vi "MAG_UI_Main.vi"() -> ()   [LabVIEW 2018]
doc: "Use this template to build a simple state machine design pattern. Each state executes code and determines which state to transition to."
uses:
  controls/MAG_UI_Data.ctl
  controls/MAG_UI_Command.ctl
  controls/MAG_Comms_State.ctl
  controls/Sensor_Data.ctl
  controls/BT_Devices.ctl
  <vilib>/Native 3D Graph/xcontrol/3DPC_SurfacePlot.xctl
  controls/MAG_UI_State.ctl
  controls/MAG_Display_State.ctl
  controls/MAG_UI_Comms_Config.ctl
  subVIs/calibration/FGVs/FGV States.ctl
panel:
  in  "Button_Sys_Check":bool
  in  "UI_Tab":T1(tab)
  out "Sensor Readings":dbl[][](array[numeric])=[[207.276, -3680.651, -5885.44], [494.158, -4382.085, -5575.68], [301.151, -4004.332, -4646.4], [401.034, -4427.145, -4646.4], [87.867, -4272.439, -4646.4], [-42.056, -4150.777, -4026.88], [-226.802, -4030.617, -3407.3599999999997], [225.3, -4882.251, -4026.88], [349.966, -3422.307, -5575.68], [254.589, -3876.662, -5575.68], [485.897, -4172.556, -4646.4], [107.393, -3751.245, -4026.88], [97.63, -4424.141, -3717.12], [-0.751, -4374.575, -4026.88], [-150.951, -3895.437, -4026.88], [-451.351, -4812.408, -4336.639999999999], [-148.698, -3219.537, -5885.44], [120.911, -4482.719, -5885.44], [-244.826, -3894.686, -4646.4], [-131.425, -3897.69, -4026.88], [-337.95, -4164.295, -4336.639999999999], [-461.865, -4094.452, -4336.639999999999], [-414.552, -3842.116, -4336.639999999999], [-774.281, -5015.929, -4646.4], [-63.084, -4473.707, -5885.44], [-47.313, -3474.126, -5265.92], [-464.869, -4331.017, 4026.88], [-458.11, -4048.641, -4646.4], [-462.616, -4204.849, -4336.639999999999], [-644.358, -4587.108, -5265.92], [-526.451, -4170.303, -4646.4], [-1116.737, -5181.9, -4956.16], [316.922, -4416.631, -5885.44], [-174.983, -3826.345, -5885.44], [-693.924, -3861.642, -4646.4], [-112.65, -4486.474, -4646.4], [-210.28, -3921.722, -4956.16], [-518.19, -4052.396, -4956.16], [-841.871, -4038.127, -4956.16], [-1354.804, -4737.308, -4956.16], [-153.204, -3745.988, -6195.2], [181.742, -3714.446, -5885.44], [0.751, 0.751, 309.76], [-799.064, -4349.041, -4956.16], [-1019.858, -4024.609, -5265.92], [-565.503, -4018.601, -5265.92], [-770.526, -4175.56, -5575.68], [-1125.749, -5006.166, -5575.68], [496.411, -4216.114, -7124.48], [-14.269, -3723.458, -6504.96], [-910.963, -4006.585, -6195.2], [-1396.86, -4133.504, -5575.68], [-1124.247, -4031.368, -4646.4], [-1948.094, -3513.929, -6195.2], [-1823.428, -3645.354, -5575.68], [-2681.07, -4476.711, -5885.44], [-389.018, -2473.794, -5575.68], [-982.308, -2724.628, -6195.2], [-1058.91, -2711.11, -5575.68], [-1121.994, -2741.15, 4956.16], [-1360.812, -3184.991, 2168.3199999999997], [-2020.941, -4083.187, -5575.68], [-1991.652, -3568.001, -5575.68], [-1966.869, -4436.908, -6195.2]]
  in  "Tab Control":enum32{"2D", "3D"}(tab)=enum."3D"
  out "Node Response":T2(graph)
  in  "Node":i32
  out "3D Graph":refnum<class "Base Datatype.lvclass">[](xcontrol)
  in  "Logfile Store":path
  in  "Get File":bool
  in  "Stop Logging":bool
  out "Elapsed Samples":i32
  in  "Log File ID":string
  out "File System Information":string
  in  "Comms Setting":enum32{"Serial", "Bluetooth"}(tab)=enum."Bluetooth"
  in  "VISA resource name":refnum<visa-resource-name>="COM11"
  in  "Serial Settings":T3={"baud rate"=115200, "data bits"=8, "parity"=enum."None", "stop bits"=10, "flow control"=0} {"flow control" items=["None"=0, "XON/XOFF"=1, "RTS/CTS"=2, "DTR/DSR"=4]; "stop bits" items=["1.0"=10, "1.5"=15, "2.0"=20]; "data bits" min=5 max=8 step=1; "baud rate" items=["75"=75, "110"=110, "134"=134, "150"=150, "300"=300, "600"=600, "1200"=1200, "1800"=1800, "2400"=2400, "4800"=4800, "7200"=7200, "9600"=9600, "14400"=14400, "19200"=19200, "28800"=28800, "38400"=38400, "56000"=56000, "57600"=57600, "115200"=115200, "128000"=128000, "230400"=230400]}
  in  "BT address":string="00:14:03:05:08:37"
  in  "BT Channel (0)":u16=1
  in  "Calibration File":string="6x0-5mm"
  out "Comm State":T4
  out "notification":T6
  out "comms":i32=1114490
  out "ui":i32=2866
  out "Comm Er":errorcluster={"status"=TRUE, "code"=1, "source"="Wait on Notification in MAG_UI_Main.vi"}
  out "Available BT Devices":T7
  in  "Discover BT Devices":bool
  in  "Button_Disconnect":bool
  in  "Button_Initialise":bool
  in  "Button_Stream":bool
  out "Status":T8={"System Version"="", "Connected"=TRUE, "Active?"=TRUE, "Streaming"=TRUE, "Logging"=FALSE}
  in  "Button_Record":bool
  in  "Button_Connect":bool
  in  "Button_Exit":bool
  # "ESCAPES"
  # "Select this tab to use Direct Bluetooth connectivity"
  # "20:16:12:12:64:24"
  # "00:06:66:8c:9e:7d"
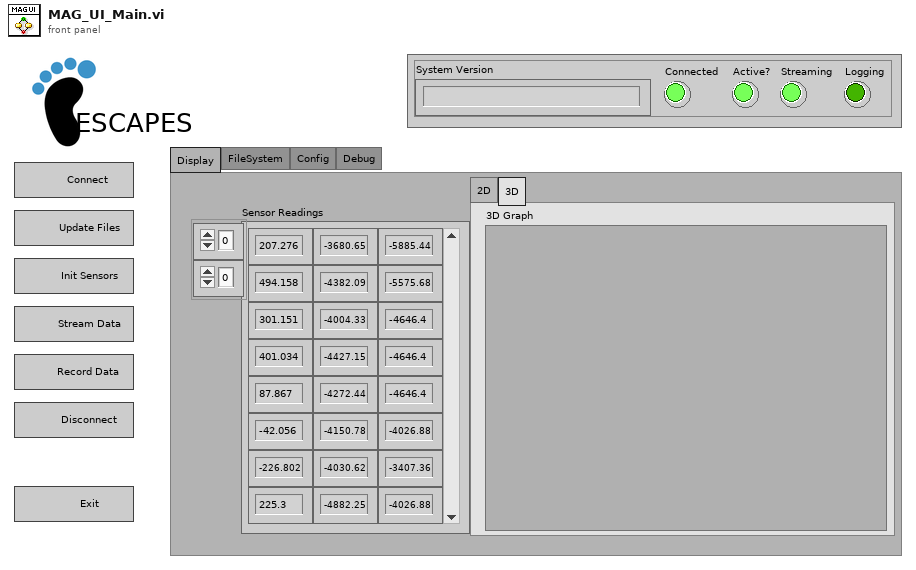
[diagram p1: front panel]
types:
  T1 = enum32{"Display", "FileSystem", "Config", "Debug"}
  T2 = cluster{"Node XYZ List[0]":dbl, "Node XYZ List[1]":dbl, "Node XYZ List[2]":dbl}
  T3 = cluster{"baud rate":u32, "data bits":u16, "parity":enum16{"None", "Odd", "Even", "Mark", "Space"}, "stop bits":u16, "flow control":u16}
  T4 = typedef "MAG_UI_Command.ctl" = cluster{"Comms_States":T5, "Parameters":string, "Clear Buffer?":bool}
  T5 = typedef "MAG_Comms_State.ctl" = enum16{"Initialize", "Wait for Event", "Connect", "Send_Com", "Rcv_TXT", "Rcv_BIN", "Rcv_FILE", "Disconnect"}
  T6 = typedef "Sensor_Data.ctl" = cluster{"Time":u32, "Data":dbl[][]}
  T7 = typedef "BT_Devices.ctl" = cluster{"Address":string, "Device Name":string}[]
  T8 = typedef "MAG_UI_Data.ctl" = cluster{"System Version":string, "Connected":bool, "Active?":bool, "Streaming":bool, "Logging":bool}
  T9 = typedef "MAG_UI_Comms_Config.ctl" = cluster{enum16{"Serial", "Bluetooth"}, "Serial Refnum":refnum<visa-resource-name>, "BT ID":refnum<k31>}
  T10 = typedef "MAG_Display_State.ctl" = enum16{"Initialise", "Display", "Exit"}
  T11 = typedef "MAG_UI_State.ctl" = enum16{"Initialize", "Wait for Event", "Com_Connect", "Com_Init_Sys", "Com_Chk_Sys", "Com_Stream", "Com_Log", "Com_Get", "Exit"}
  T12 = typedef "FGV States.ctl" = enum16{"Get", "Set", "Reset"}
  T13 = cluster{cluster{dbl[][], "Array":dbl[][]}, cluster{dbl[][], "Array":dbl[][]}, cluster{dbl[][], "Array":dbl[][]}, cluster{dbl[][], "Array":dbl[][]}}
  T14 = cluster{cluster{dbl[][], "Array":dbl[][]}, cluster{dbl[][], "Array":dbl[][]}, cluster{dbl[][], "Array":dbl[][]}, cluster{dbl[][], "Array":dbl[][]}}[]
  T15 = cluster{"Mag_GRID[0]":dbl, "Mag_GRID[1]":dbl, "Mag_GRID[2]":dbl}
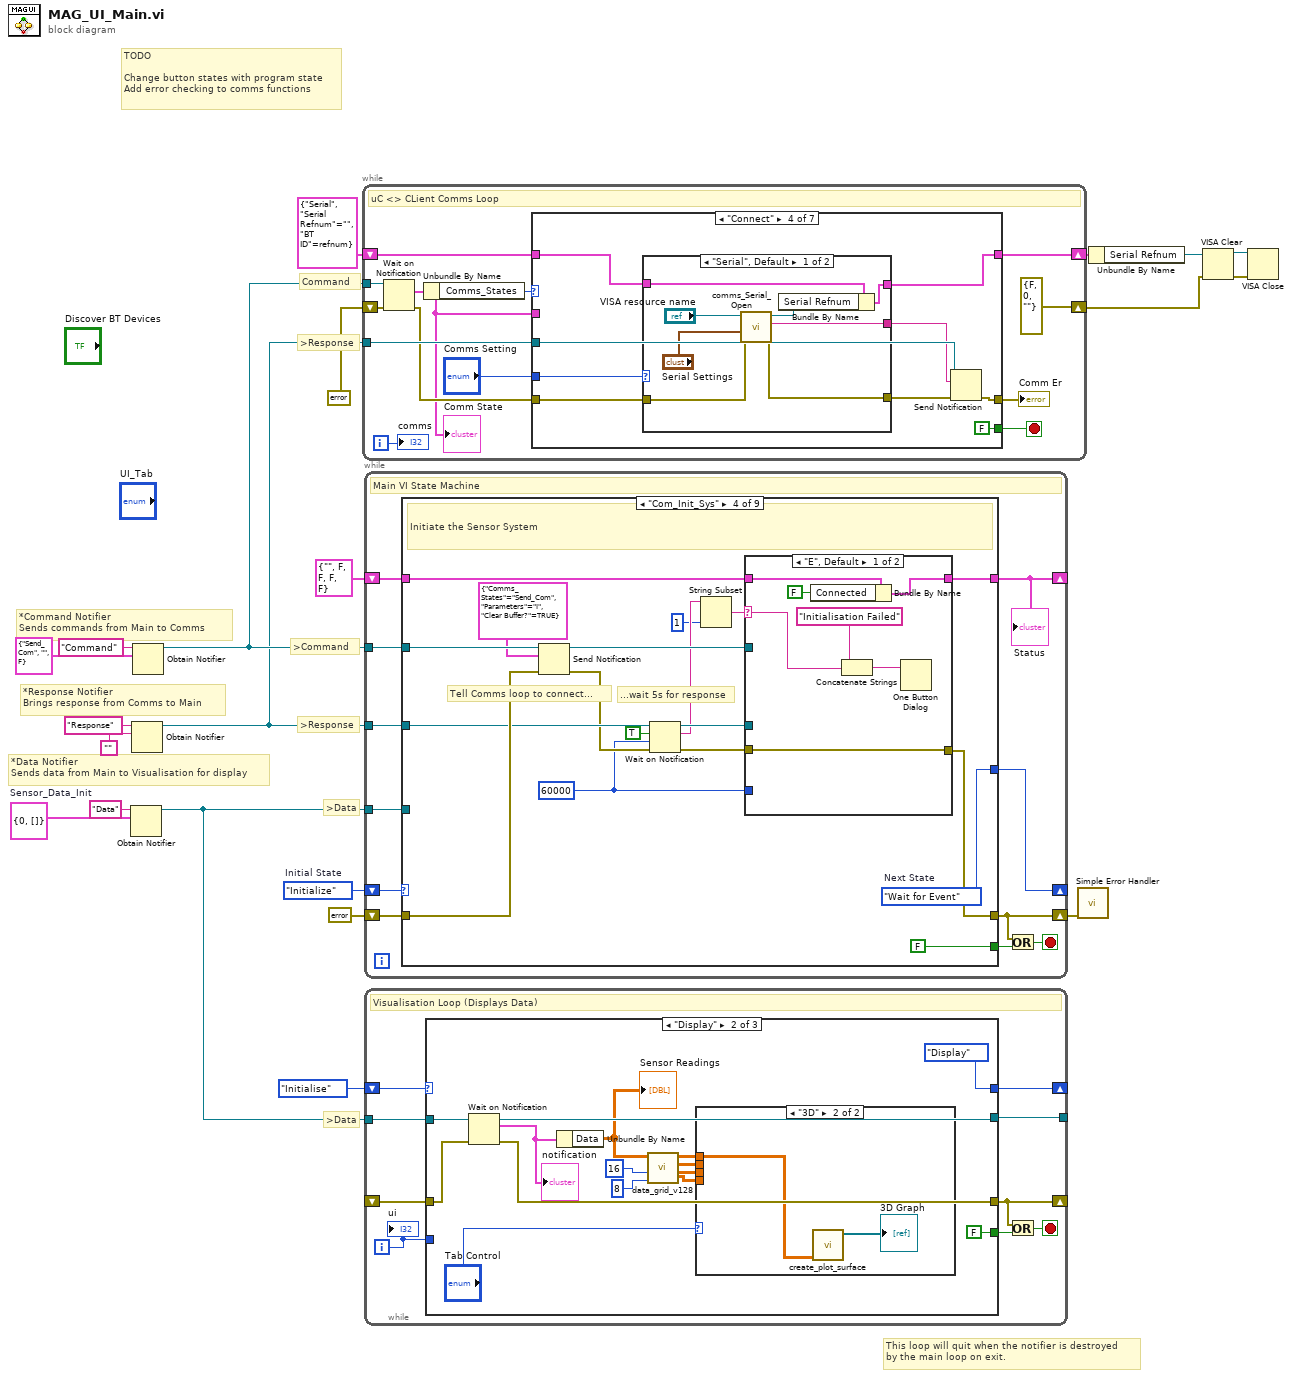
[diagram p0: block diagram]
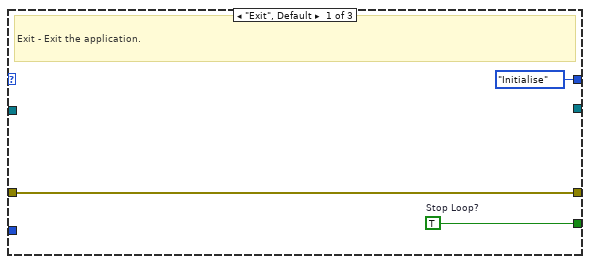
[diagram p2: hidden frame]
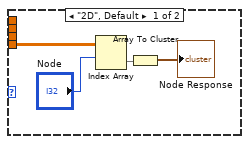
[diagram p3: hidden frame]
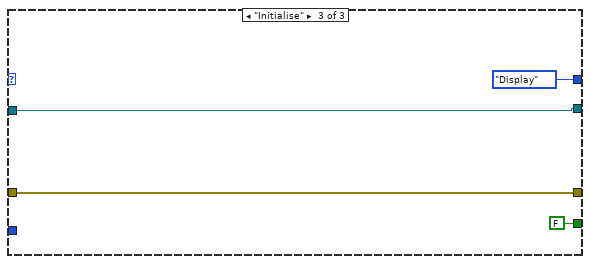
[diagram p4: hidden frame]
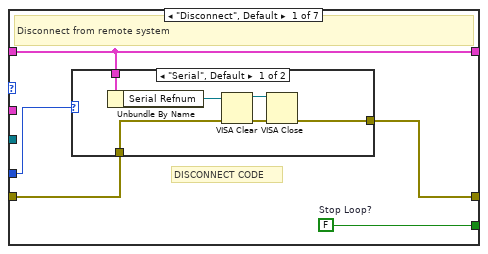
[diagram p5: hidden frame]
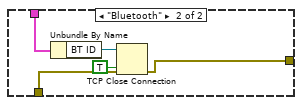
[diagram p6: hidden frame]
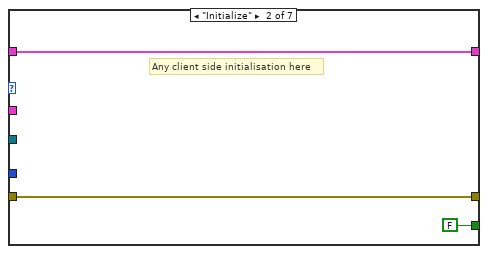
[diagram p7: hidden frame]
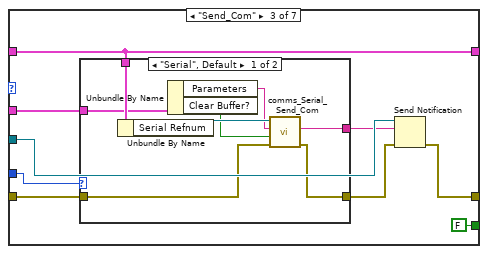
[diagram p8: hidden frame]
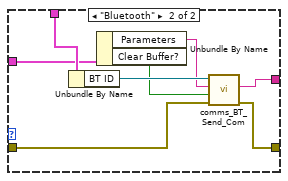
[diagram p9: hidden frame]
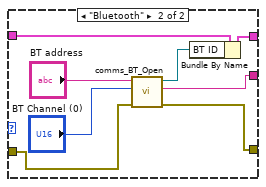
[diagram p10: hidden frame]
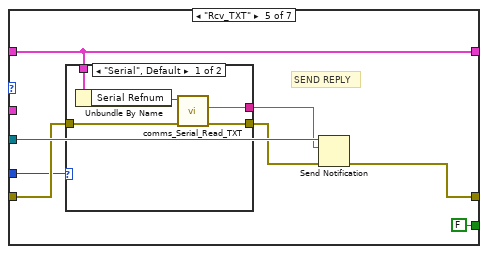
[diagram p11: hidden frame]
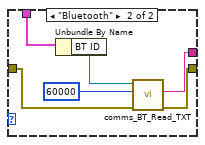
[diagram p12: hidden frame]
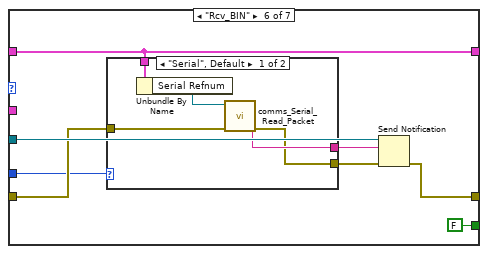
[diagram p13: hidden frame]
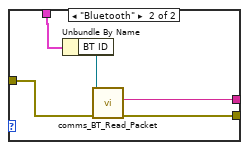
[diagram p14: hidden frame]
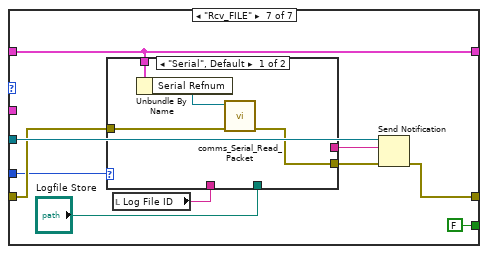
[diagram p15: hidden frame]
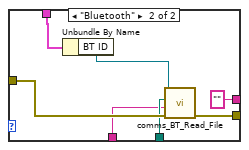
[diagram p16: hidden frame]
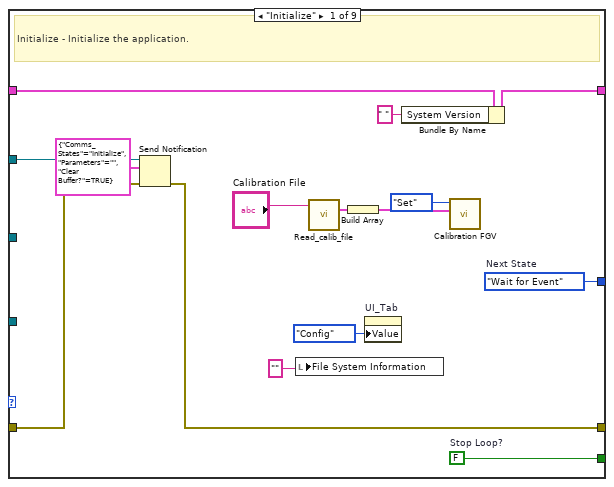
[diagram p17: hidden frame]
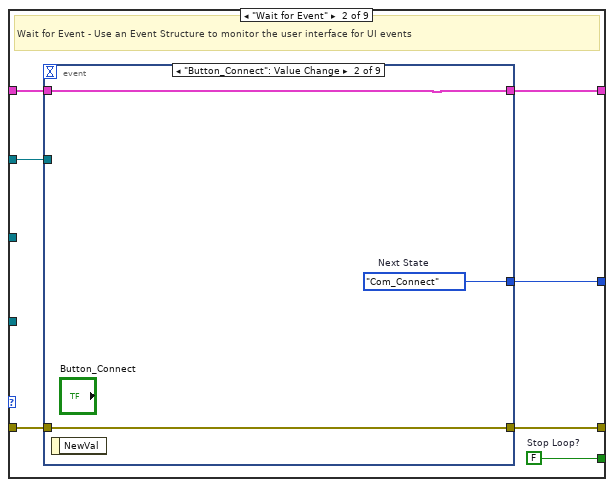
[diagram p18: hidden frame]
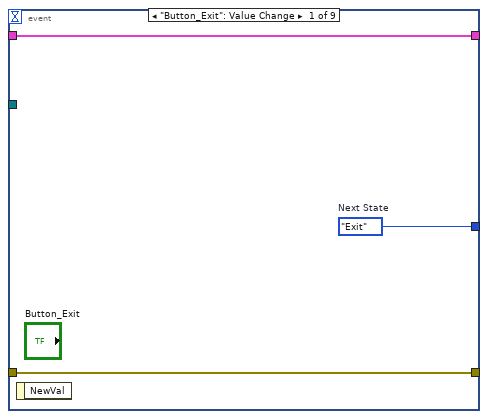
[diagram p19: hidden frame]
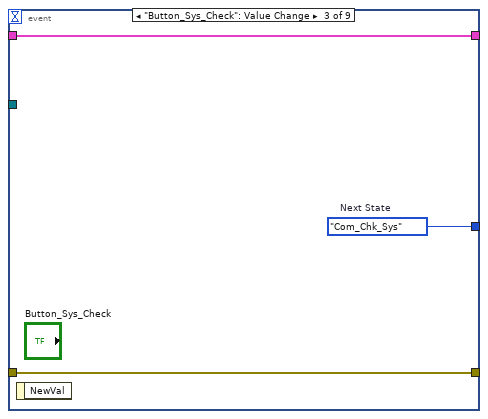
[diagram p20: hidden frame]
diagram:
  w10 = T6 {"Time"=0, "Data"=[]}  # Sensor_Data_Init
  w21 = MAG_UI_State."Initialize"  # Initial State
  # "TODO\n\nChange button states with program state\nAdd error checking to comms functions"
  # "This loop will quit when the notifier is destroyed\nby the main loop on exit."
  # ">Data"
  # ">Data"
  # ">Response"
  # ">Response"
  # ">Command"
  # "*Data Notifier\nSends data from Main to Visualisation for display"
  # "*Response Notifier\nBrings response from Comms to Main"
  # "*Command Notifier\nSends commands from Main to Comms"
  # "Command"
  n1 = Obtain Notifier(name (unnamed)="Data", notification data type=w10) -> (notifier out=w12:refnum<notifier>)  [unwired: 2 in, 2 out]
  n2 = Obtain Notifier(name (unnamed)="Response", notification data type="") -> (notifier out=w11:refnum<notifier>)  [unwired: 2 in, 2 out]
  n3 = Obtain Notifier(name (unnamed)="Command", notification data type=T4 {"Comms_States"=enum."Send_Com", "Parameters"="", "Clear Buffer?"=FALSE}) -> (notifier out=w15:refnum<notifier>)  [unwired: 2 in, 2 out]
  n4 = while {
    shift-right: [errorcluster {"status"=FALSE, "code"=0, "source"=""} ("error constant")] -> w1
    shift-left: errorcluster {"status"=FALSE, "code"=0, "source"=""} ("error constant") -> [w30]
    tunnel: w15 -> [w32]
    tunnel: w11 -> [w34]
    shift-right: [w27] -> w2
    shift-left: T9 {enum."Serial", "Serial Refnum"="", "BT ID"=refnum} -> [w28]
    i -> [w26]
    stop <- w24 stop-if-true
    # "uC <> CLient Comms Loop"
    n5 = Wait on Notification(notifier=w32, error in (no error)=w30) -> (notification=w25:T4, error out=w29:errorcluster)  [unwired: 2 in, 2 out]
    "Comm State" <- w25
    n6 = Unbundle By Name(w25) -> ("Comms_States"=w31:T5)
    n7 = case shown="\"Connect\"" w31 {
      tunnel: [w39 FALSE ("Stop Loop?") FALSE ("Stop Loop?") FALSE ("Stop Loop?") FALSE ("Stop Loop?") FALSE ("Stop Loop?") FALSE ("Stop Loop?")] -> w24
      tunnel: w29 -> [w38 w52 w57 w81 w107 w125 w145]
      tunnel: [w37 w52 w61 w87 w110 w129 w149] -> w33
      tunnel: w34 -> [_ _ w62 w85 w111 w128 w148]
      tunnel: w28 -> [w36 w51 w58 w83 w108 w126 w146]
      tunnel: [w36 w51 w58 w82 w108 w126 w146] -> w27
      tunnel: w25 -> [_ _ w55 _ _ _ _]
      tunnel: "Comms Setting" -> [w35 _ w54 w79 w104 w123 w143]
      frame "Disconnect", Default {
        w39 = FALSE  # Stop Loop?
        # "DISCONNECT CODE"
        # "Disconnect from remote system"
        n8 = case shown="\"Serial\", Default" w35 {
          tunnel: w38 -> [w42 w48]
          tunnel: [w41 w47] -> w37
          tunnel: w36 -> [w40 w50]
          frame "Serial", Default {
            n9 = Unbundle By Name(w40) -> ("Serial Refnum"=w45:refnum<visa-resource-name>)
            n10 = VISA Clear(VISA resource name=w45, error in (no error)=w42) -> (VISA resource name out=w43:refnum<visa-resource-name>, error out=w44:errorcluster)
            n11 = VISA Close(VISA resource name=w43, error in (no error)=w44) -> (error out=w41:errorcluster)
          }
          frame "Bluetooth" {
            n12 = Unbundle By Name(w50) -> ("BT ID"=w49:refnum<k31>)
            n13 = TCP Close Connection(connection ID=w49, abort (F)=TRUE, error in (no error)=w48) -> (error out=w47:errorcluster)  [unwired: 1 out]
          }
        }
      }
      frame "Initialize" {
        # "Any client side initialisation here"
      }
      frame "Send_Com" {
        n14 = case shown="\"Serial\", Default" w54 {
          tunnel: [w69 w71] -> w59
          tunnel: w58 -> [w68 w78]
          tunnel: w57 -> [w67 w76]
          tunnel: [w66 w75] -> w56
          tunnel: w55 -> [w64 w77]
          frame "Serial", Default {
            n15 = Unbundle By Name(w68) -> ("Serial Refnum"=w70:refnum<visa-resource-name>)
            n16 = Unbundle By Name(w64) -> ("Parameters"=w63:string, "Clear Buffer?"=w65:bool)
            n17 = call "comms_Serial_Send_Com.vi"("error in"=w67, "Buffer Clear?"=w65, "Command"=w63, "VISA resource in"=w70) -> ("error out"=w66:errorcluster, "Response"=w69:string)  [unwired: 5 in, 1 out]
          }
          frame "Bluetooth" {
            n18 = Unbundle By Name(w78) -> ("BT ID"=w74:refnum<k31>)
            n19 = Unbundle By Name(w77) -> ("Parameters"=w73:string, "Clear Buffer?"=w72:bool)
            n20 = call "comms_BT_Send_Com.vi"("error in"=w76, "Buffer Clear?"=w72, "Command"=w73, "connection ID"=w74) -> ("error out"=w75:errorcluster, "Response"=w71:string)  [unwired: 5 in, 1 out]
          }
        }
        n21 = Send Notification(notification=w59, notifier=w62, error in (no error)=w56) -> (error out=w61:errorcluster)  [unwired: 1 out]
      }
      frame "Connect" {
        n22 = case shown="\"Serial\", Default" w79 {
          tunnel: [w89 w100] -> w84
          tunnel: w83 -> [w93 w99]
          tunnel: [w91 w97] -> w82
          tunnel: w81 -> [w90 w101]
          tunnel: [w88 w96] -> w80
          frame "Serial", Default {
            n23 = call "comms_Serial_Open.vi"("error in (no error)"=w90, "Serial Settings in"="Serial Settings", "VISA Refnum in"="VISA resource name") -> ("error out"=w89:errorcluster, "Data Out"=w88:string, "VISA Refnum out"=w92:refnum<visa-resource-name>)  [unwired: 6 in]
            n24 = Bundle By Name(cluster=w93, "Serial Refnum"=w92) -> (w91:T9)
          }
          frame "Bluetooth" {
            n25 = call "comms_BT_Open.vi"("error in (no error)"=w101, "BT Channel (0)"="BT Channel (0)", "BT address"="BT address") -> ("error out"=w100:errorcluster, "Response"=w96:string, "Bluetooth Network Connection out"=w98:refnum<k31>)  [unwired: 6 in]
            n26 = Bundle By Name(cluster=w99, "BT ID"=w98) -> (w97:T9)
          }
        }
        n27 = Send Notification(notification=w80, notifier=w85, error in (no error)=w84) -> (error out=w87:errorcluster)  [unwired: 1 out]
      }
      frame "Rcv_TXT" {
        # "SEND REPLY"
        n28 = case shown="\"Serial\", Default" w104 {
          tunnel: w108 -> [w116 w122]
          tunnel: w107 -> [w114 w118]
          tunnel: [w113 w119] -> w106
          tunnel: [w112 w120] -> w105
          frame "Serial", Default {
            n29 = Unbundle By Name(w116) -> ("Serial Refnum"=w115:refnum<visa-resource-name>)
            n30 = call "comms_Serial_Read_TXT.vi"("error in"=w114, "VISA resource in"=w115) -> ("error out"=w113:errorcluster, "Data Out"=w112:string)  [unwired: 6 in, 2 out]
          }
          frame "Bluetooth" {
            n31 = Unbundle By Name(w122) -> ("BT ID"=w121:refnum<k31>)
            n32 = call "comms_BT_Read_TXT.vi"("error in"=w118, "timeout ms (25000)"=60000, "connection ID"=w121) -> ("error out"=w119:errorcluster, "Data Out"=w120:string)  [unwired: 5 in, 2 out]
          }
        }
        n33 = Send Notification(notification=w105, notifier=w111, error in (no error)=w106) -> (error out=w110:errorcluster)  [unwired: 1 out]
      }
      frame "Rcv_BIN" {
        n34 = case shown="\"Serial\", Default" w123 {
          tunnel: [w135 w136] -> w127
          tunnel: w126 -> [w133 w140]
          tunnel: w125 -> [w132 w138]
          tunnel: [w131 w137] -> w124
          frame "Serial", Default {
            n35 = Unbundle By Name(w133) -> ("Serial Refnum"=w134:refnum<visa-resource-name>)
            n36 = call "comms_Serial_Read_Packet.vi"("error in"=w132, "VISA resource in"=w134) -> ("error out"=w131:errorcluster, "Data Out"=w135:string)  [unwired: 6 in, 2 out]
          }
          frame "Bluetooth" {
            n37 = Unbundle By Name(w140) -> ("BT ID"=w139:refnum<k31>)
            n38 = call "comms_BT_Read_Packet.vi"("error in"=w138, "connection ID"=w139) -> ("error out"=w137:errorcluster, "Data Out"=w136:string)  [unwired: 7 in, 1 out]
          }
        }
        n39 = Send Notification(notification=w127, notifier=w128, error in (no error)=w124) -> (error out=w129:errorcluster)  [unwired: 1 out]
      }
      frame "Rcv_FILE" {
        n40 = local read "Log File ID"() -> (w141:string)
        n41 = case shown="\"Serial\", Default" w143 {
          tunnel: [_ "" ("source")] -> w147
          tunnel: w146 -> [w153 w161]
          tunnel: w145 -> [w152 w159]
          tunnel: [w151 w158] -> w144
          tunnel: "Logfile Store" -> [_ w156]
          tunnel: w141 -> [_ w155]
          frame "Serial", Default {
            n42 = Unbundle By Name(w153) -> ("Serial Refnum"=w154:refnum<visa-resource-name>)
            n43 = call "comms_Serial_Read_Packet.vi"("error in"=w152, "VISA resource in"=w154) -> ("error out"=w151:errorcluster)  [unwired: 6 in, 3 out]
          }
          frame "Bluetooth" {
            n44 = Unbundle By Name(w161) -> ("BT ID"=w160:refnum<k31>)
            n45 = call "comms_BT_Read_File.vi"("error in"=w159, "filename"=w155, "file path (use dialog)"=w156, "connection ID"=w160) -> ("error out"=w158:errorcluster)  [unwired: 6 in, 1 out]
          }
        }
        n46 = Send Notification(notification=w147, notifier=w148, error in (no error)=w144) -> (error out=w149:errorcluster)  [unwired: 1 out]
      }
    }
    "Comm Er" <- w33
    "comms" <- w26
  }
  n47 = while {
    shift-right: [w171] -> _
    shift-left: w21 -> [w172]
    shift-right: [w162] -> _
    shift-left: T8 {"System Version"="", "Connected"=FALSE, "Active?"=FALSE, "Streaming"=FALSE, "Logging"=FALSE} ("Data") -> [w170]
    shift-right: [w166] -> w18
    shift-left: errorcluster {"status"=FALSE, "code"=0, "source"=""} ("error constant") -> [w169]
    tunnel: w15 -> [w165]
    tunnel: w11 -> [w164]
    tunnel: w12 -> [w163]
    stop <- w167 stop-if-true
    # "Main VI State Machine"
    n48 = case shown="\"Com_Init_Sys\"" w172 {
      tunnel: [w187 w194 w248 w267 w305 w340 w376 w420 w462] -> w171
      tunnel: [w186 w193 FALSE ("Stop Loop?") FALSE ("Stop Loop?") FALSE ("Stop Loop?") FALSE ("Stop Loop?") FALSE ("Stop Loop?") FALSE ("Stop Loop?") w460] -> w168
      tunnel: w170 -> [w185 w192 w240 w271 w308 w344 w380 w423 w461]
      tunnel: [w184 w191 w239 w270 w307 w343 w379 w422 w461] -> w162
      tunnel: w169 -> [w180 w190 w245 w274 w311 w347 w383 w426 w456]
      tunnel: [w179 w189 w242 w264 w302 w337 w373 w417 w455] -> w166
      tunnel: w165 -> [w182 w188 w246 w275 w312 w348 w384 w427 w459]
      tunnel: w164 -> [_ _ w244 w273 w310 w346 w382 w425 w453]
      tunnel: w163 -> [_ _ _ _ _ _ w369 w413 w452]
      frame "Initialize" {
        w186 = FALSE  # Stop Loop?
        w187 = MAG_UI_State."Wait for Event"  # Next State
        # "Initialize - Initialize the application."
        n49 = Send Notification(notification=T4 {"Comms_States"=enum."Initialize", "Parameters"="", "Clear Buffer?"=TRUE}, notifier=w182, error in (no error)=w180) -> (error out=w179:errorcluster)  [unwired: 1 out]
        n50 = local write "File System Information"("" ("File System Information")) -> ()
        n51 = call "Read_calib_file.vi"("string"="Calibration File") -> ("output cluster"=w175:T13)  [unwired: 6 in, 4 out]
        n52 = Build Array(w175) -> (w174:T14)
        n53 = property on="UI_Tab" class="TabCtl (strict)"("Value"=T1."Config" ("UI_Tab")) -> ()  [unwired: 2 in, 2 out]
        n54 = Bundle By Name(cluster=w185, "System Version"=" ") -> (w184:T8)
        n55 = call "Calibration FGV.vi"("Calib in"=w174, "FGV States"=FGV_States."Set") -> ()  [unwired: 9 in, 1 out]
      }
      frame "Wait for Event" {
        w193 = FALSE  # Stop Loop?
        # "Wait for Event - Use an Event Structure to monitor the user interface for UI events"
        n56 = event shown="[1] \"Button_Connect\": Value Change" {
          selector: _ -> [_ _ _ _ _ _ _ _ _]
          dyn-events: _ -> [_ _ _ _ _ _ _ _ _]
          timeout: _ -> [_ _ _ _ _ _ _ _ _]
          tunnel: [w197 w200 w203 MAG_UI_State."Com_Init_Sys" ("Next State") MAG_UI_State."Com_Stream" ("Next State") MAG_UI_State."Wait for Event" ("Next State") MAG_UI_State."Com_Log" ("Next State") MAG_UI_State."Com_Get" ("Next State") MAG_UI_State."Wait for Event" ("Next State")] -> w194
          tunnel: w192 -> [w196 w198 w201 w206 w209 w215 w217 w223 w230]
          tunnel: [w196 w198 w201 w206 w208 w215 w216 w223 w229] -> w191
          tunnel: w190 -> [w195 w199 w202 w205 w211 w214 w220 w222 w232]
          tunnel: [w195 w199 w202 w205 w211 w214 w220 w222 w226] -> w189
          tunnel: w188 -> [_ _ _ _ _ _ _ _ w233]
          event "Button_Exit": Value Change {
            w197 = MAG_UI_State."Exit"  # Next State
            n57 = event-data() -> ()  [unwired: 1 in, 1 out]
          }
          event "Button_Connect": Value Change {
            w200 = MAG_UI_State."Com_Connect"  # Next State
            n58 = event-data() -> ()  [unwired: 1 in, 1 out]
          }
          event "Button_Sys_Check": Value Change {
            w203 = MAG_UI_State."Com_Chk_Sys"  # Next State
            n59 = event-data() -> ()  [unwired: 1 in, 1 out]
          }
          event "Button_Initialise": Value Change {
            n60 = event-data() -> ()  [unwired: 1 in, 1 out]
          }
          event "Button_Stream": Value Change {
            n61 = event-data() -> ()  [unwired: 1 in, 1 out]
            n62 = Bundle By Name(cluster=w209, "Streaming"=TRUE) -> (w208:T8)
          }
          event "Discover BT Devices": Value Change {
            n63 = event-data() -> ()  [unwired: 1 in, 1 out]
            n64 = call "BT_Discover.vi"() -> ("Active_BT_Devices"=→"Available BT Devices":T7)  [unwired: 11 in]
          }
          event "Button_Record": Value Change {
            n65 = event-data() -> ()  [unwired: 1 in, 1 out]
            n66 = Bundle By Name(cluster=w217, "Logging"=TRUE ("Streaming")) -> (w216:T8)
          }
          event "Get File": Value Change {
            n67 = event-data() -> ()  [unwired: 1 in, 1 out]
          }
          event "Button_Disconnect": Value Change {
            n68 = event-data() -> ()  [unwired: 1 in, 1 out]
            n69 = Send Notification(notification=T4 {"Comms_States"=enum."Send_Com", "Parameters"="X", "Clear Buffer?"=TRUE}, notifier=w233, error in (no error)=w232) -> (notifier out=w224:refnum<notifier>, error out=w227:errorcluster)
            n70 = Send Notification(notification=T4 {"Comms_States"=enum."Disconnect", "Parameters"="X", "Clear Buffer?"=TRUE}, notifier=w224, error in (no error)=w227) -> (error out=w226:errorcluster)  [unwired: 1 out]
            n71 = Bundle By Name(cluster=w230, "System Version"="") -> (w229:T8)
          }
        }
      }
      frame "Com_Connect" {
        w248 = MAG_UI_State."Wait for Event"  # Next State
        # "...wait 5s for response"
        # "Tell Comms loop to connect..."
        # "Connect to the System"
        n72 = Send Notification(notification=T4 {"Comms_States"=enum."Connect", "Parameters"="", "Clear Buffer?"=TRUE}, notifier=w246, error in (no error)=w245) -> (error out=w243:errorcluster)  [unwired: 1 out]
        n73 = Wait on Notification(notifier=w244, timeout in ms (-1)=5000, error in (no error)=w243) -> (notification=w235:string, error out=w242:errorcluster)  [unwired: 1 in, 2 out]
        n74 = String Subset(string=w235, length (rest)=1 ("offset (0)")) -> (substring=w237:string)  [unwired: 1 in]
        n75 = case shown="\"!\", Default" w237 {
          tunnel: w240 -> [w252 w256]
          tunnel: [w251 w255] -> w239
          tunnel: w235 -> [w249 w253]
          frame "!", Default {
            n76 = Bundle By Name(cluster=w252, "Connected"=TRUE, "System Version"=w249) -> (w251:T8)
          }
          frame "E" {
            n77 = Bundle By Name(cluster=w256, "Connected"=FALSE) -> (w255:T8)
            n78 = Concatenate Strings("Connection Error", w253) -> (w258:string)
            n79 = One Button Dialog(message=w258) -> ()  [unwired: 1 in, 1 out]
          }
        }
      }
      frame "Com_Init_Sys" {
        w267 = MAG_UI_State."Wait for Event"  # Next State
        w266 = 60000 ("timeout in ms (-1)")
        # "...wait 5s for response"
        # "Tell Comms loop to connect..."
        # "Initiate the Sensor System"
        n80 = Send Notification(notification=T4 {"Comms_States"=enum."Send_Com", "Parameters"="I", "Clear Buffer?"=TRUE}, notifier=w275, error in (no error)=w274) -> (notifier out=w268:refnum<notifier>, error out=w272:errorcluster)
        n81 = Wait on Notification(notifier=w273, ignore previous (F)=TRUE, timeout in ms (-1)=w266, error in (no error)=w272) -> (notifier out=w263:refnum<notifier>, notification=w260:string, error out=w265:errorcluster)  [unwired: 1 out]
        n82 = String Subset(string=w260, length (rest)=1 ("offset (0)")) -> (substring=w261:string)  [unwired: 1 in]
        n83 = case shown="\"E\", Default" w261 {
          selector: w261 -> [w281 _]
          tunnel: w271 -> [w280 w287]
          tunnel: [w279 w286] -> w270
          tunnel: w268 -> [_ w294]
          tunnel: w266 -> [_ w293]
          tunnel: w265 -> [w277 w292]
          tunnel: [w277 w290] -> w264
          tunnel: w263 -> [_ w289]
          frame "E", Default {
            n84 = Bundle By Name(cluster=w280, "Connected"=FALSE) -> (w279:T8)
            n85 = Concatenate Strings("Initialisation Failed", w281) -> (w283:string)
            n86 = One Button Dialog(message=w283) -> ()  [unwired: 1 in, 1 out]
          }
          frame "i" {
            n87 = Send Notification(notification=T4 {"Comms_States"=enum."Rcv_TXT", "Parameters"="", "Clear Buffer?"=FALSE}, notifier=w294, error in (no error)=w292) -> (error out=w291:errorcluster)  [unwired: 1 out]
            n88 = Bundle By Name(cluster=w287, "Active?"=TRUE) -> (w286:T8)
            n89 = Wait on Notification(notifier=w289, ignore previous (F)=TRUE, timeout in ms (-1)=w293, error in (no error)=w291) -> (notification=w284:string, error out=w290:errorcluster)  [unwired: 2 out]
            n90 = One Button Dialog(message=w284) -> ()  [unwired: 1 in, 1 out]
          }
        }
      }
      frame "Com_Get" {
        w305 = MAG_UI_State."Wait for Event"  # Next State
        w304 = 120000 ("timeout in ms (-1)")
        # "...wait 5s for response"
        # "Tell Comms loop to connect..."
        # "Initiate the Sensor System"
        n91 = Send Notification(notification=T4 {"Comms_States"=enum."Send_Com", "Parameters"="G", "Clear Buffer?"=TRUE}, notifier=w312, error in (no error)=w311) -> (notifier out=w306:refnum<notifier>, error out=w309:errorcluster)
        n92 = Wait on Notification(notifier=w310, ignore previous (F)=TRUE, timeout in ms (-1)=w304, error in (no error)=w309) -> (notifier out=w301:refnum<notifier>, notification=w298:string, error out=w303:errorcluster)  [unwired: 1 out]
        n93 = String Subset(string=w298, length (rest)=1 ("offset (0)")) -> (substring=w299:string)  [unwired: 1 in]
        n94 = case shown="\"g\"" w299 {
          selector: w299 -> [w318 _]
          tunnel: w308 -> [w317 w324]
          tunnel: [w316 w323] -> w307
          tunnel: w306 -> [_ w330]
          tunnel: w304 -> [_ _]
          tunnel: w303 -> [w314 w329]
          tunnel: [w314 w327] -> w302
          tunnel: w301 -> [_ w326]
          frame "E", Default {
            n95 = Bundle By Name(cluster=w317, "Connected"=FALSE) -> (w316:T8)
            n96 = Concatenate Strings("Initialisation Failed", w318) -> (w320:string)
            n97 = One Button Dialog(message=w320) -> ()  [unwired: 1 in, 1 out]
          }
          frame "g" {
            n98 = Send Notification(notification=T4 {"Comms_States"=enum."Rcv_FILE", "Parameters"="", "Clear Buffer?"=FALSE}, notifier=w330, error in (no error)=w329) -> (error out=w328:errorcluster)  [unwired: 1 out]
            n99 = Bundle By Name(cluster=w324, "Active?"=TRUE) -> (w323:T8)
            n100 = Wait on Notification(notifier=w326, ignore previous (F)=TRUE, timeout in ms (-1)=-1, error in (no error)=w328) -> (error out=w327:errorcluster)  [unwired: 3 out]
          }
        }
      }
      frame "Com_Chk_Sys" {
        w340 = MAG_UI_State."Wait for Event"  # Next State
        w339 = 25000 ("timeout in ms (-1)")
        # "...wait 5s for response"
        # "Tell Comms loop to connect..."
        # "Check the System Status"
        n101 = Send Notification(notification=T4 {"Comms_States"=enum."Send_Com", "Parameters"="C", "Clear Buffer?"=TRUE}, notifier=w348, error in (no error)=w347) -> (notifier out=w341:refnum<notifier>, error out=w345:errorcluster)
        n102 = Wait on Notification(notifier=w346, ignore previous (F)=TRUE, timeout in ms (-1)=w339, error in (no error)=w345) -> (notifier out=w336:refnum<notifier>, notification=w333:string, error out=w338:errorcluster)  [unwired: 1 out]
        n103 = String Subset(string=w333, length (rest)=1 ("offset (0)")) -> (substring=w334:string)  [unwired: 1 in]
        n104 = case shown="\"c\"" w334 {
          selector: w334 -> [w354 _]
          tunnel: w344 -> [w353 w366]
          tunnel: [w352 w366] -> w343
          tunnel: w341 -> [_ w364]
          tunnel: w339 -> [_ w363]
          tunnel: w338 -> [w350 w362]
          tunnel: [w350 w360] -> w337
          tunnel: w336 -> [_ w359]
          frame "E", Default {
            n105 = Bundle By Name(cluster=w353, "Connected"=FALSE) -> (w352:T8)
            n106 = Concatenate Strings("Initialisation Failed", w354) -> (w356:string)
            n107 = One Button Dialog(message=w356) -> ()  [unwired: 1 in, 1 out]
          }
          frame "c" {
            n108 = Send Notification(notification=T4 {"Comms_States"=enum."Rcv_TXT", "Parameters"="", "Clear Buffer?"=FALSE}, notifier=w364, error in (no error)=w362) -> (error out=w361:errorcluster)  [unwired: 1 out]
            n109 = Wait on Notification(notifier=w359, ignore previous (F)=TRUE, timeout in ms (-1)=w363, error in (no error)=w361) -> (notification=→"File System Information":string, error out=w360:errorcluster)  [unwired: 2 out]
          }
        }
      }
      frame "Com_Stream" {
        w376 = MAG_UI_State."Wait for Event"  # Next State
        w375 = 60000 ("timeout in ms (-1)")
        # "...wait for response"
        # "Tell Comms loop to connect..."
        # "Check the System Status"
        n110 = Send Notification(notification=T4 {"Comms_States"=enum."Send_Com", "Parameters"="S>", "Clear Buffer?"=TRUE}, notifier=w384, error in (no error)=w383) -> (notifier out=w377:refnum<notifier>, error out=w381:errorcluster)
        n111 = Wait on Notification(notifier=w382, ignore previous (F)=TRUE, timeout in ms (-1)=w375, error in (no error)=w381) -> (notifier out=w372:refnum<notifier>, notification=w367:string, error out=w374:errorcluster)  [unwired: 1 out]
        n112 = String Subset(string=w367, length (rest)=1 ("offset (0)")) -> (substring=w370:string)  [unwired: 1 in]
        n113 = case shown="\"s\"" w370 {
          tunnel: w380 -> [w390 w396]
          tunnel: [w389 w394] -> w379
          tunnel: w377 -> [_ w402]
          tunnel: w375 -> [_ w401]
          tunnel: w374 -> [w387 w400]
          tunnel: [w387 w399] -> w373
          tunnel: w372 -> [_ w398]
          tunnel: w369 -> [_ w397]
          tunnel: w367 -> [w386 _]
          frame "E", Default {
            n114 = Bundle By Name(cluster=w390, "Connected"=FALSE) -> (w389:T8)
            n115 = Concatenate Strings("Stream Failed", w386) -> (w392:string)
            n116 = One Button Dialog(message=w392) -> ()  [unwired: 1 in, 1 out]
          }
          frame "s" {
            n117 = Bundle By Name(cluster=w396, "Streaming"=FALSE) -> (w394:T8)
            n118 = call "stream_data.vi"("timeout in ms (-1)"=w401, "error in (no error)"=w400, "Display"=w397, "Response"=w398, "Command"=w402) -> ("error out"=w399:errorcluster)  [unwired: 6 in]
            n119 = property on="UI_Tab" class="TabCtl (strict)"("Value"=T1."Display" ("UI_Tab")) -> ()  [unwired: 2 in, 2 out]
          }
        }
      }
      frame "Com_Log" {
        w420 = MAG_UI_State."Wait for Event"  # Next State
        w419 = 60000 ("timeout in ms (-1)")
        # "Send 3 char\nfile ID for logging"
        # "...wait for response"
        # "Tell Comms loop to connect..."
        # "Check the System Status"
        n120 = String Subset(string="Log File ID", length (rest)=3 ("length (rest)")) -> (substring=w405:string)  [unwired: 1 in]
        n121 = Concatenate Strings("L" ("Parameters"), w405) -> (w408:string)
        n122 = Bundle By Name(cluster=T4 {"Comms_States"=enum."Send_Com", "Parameters"="L", "Clear Buffer?"=TRUE}, "Parameters"=w408) -> (w409:T4)
        n123 = Send Notification(notification=w409, notifier=w427, error in (no error)=w426) -> (notifier out=w421:refnum<notifier>, error out=w424:errorcluster)
        n124 = Wait on Notification(notifier=w425, ignore previous (F)=TRUE, timeout in ms (-1)=w419, error in (no error)=w424) -> (notifier out=w416:refnum<notifier>, notification=w411:string, error out=w418:errorcluster)  [unwired: 1 out]
        n125 = property on="UI_Tab" class="TabCtl (strict)"("Value"=T1."FileSystem" ("UI_Tab")) -> ()  [unwired: 2 in, 2 out]
        n126 = String Subset(string=w411, length (rest)=1 ("offset (0)")) -> (substring=w414:string)  [unwired: 1 in]
        n127 = case shown="\"l\"" w414 {
          tunnel: w423 -> [w433 w448]
          tunnel: [w432 w446] -> w422
          tunnel: w421 -> [_ w443]
          tunnel: w419 -> [_ w441]
          tunnel: w418 -> [w430 w442]
          tunnel: [w430 w439] -> w417
          tunnel: w416 -> [_ w440]
          tunnel: w413 -> [_ _]
          tunnel: w411 -> [w429 _]
          frame "E", Default {
            n128 = Bundle By Name(cluster=w433, "Connected"=FALSE) -> (w432:T8)
            n129 = Concatenate Strings("Logging Failed", w429) -> (w435:string)
            n130 = One Button Dialog(message=w435) -> ()  [unwired: 1 in, 1 out]
          }
          frame "l" {
            n131 = while {
              tunnel: ["Stop Logging"] -> w436
              i -> [w450]
              stop <- "Stop Logging" stop-if-true
              n132 = Wait Until Next ms Multiple(millisecond multiple=u32 10) -> ()  [unwired: 1 out]
              "Elapsed Samples" <- w450
            }
            n133 = Bundle By Name(cluster=T4 {"Comms_States"=enum."Send_Com", "Parameters"=".", "Clear Buffer?"=TRUE}, "Clear Buffer?"=w436) -> (w437:T4)
            n134 = Send Notification(notification=w437, notifier=w443, error in (no error)=w442) -> (error out=w444:errorcluster)  [unwired: 1 out]
            n135 = Bundle By Name(cluster=w448, "Logging"=FALSE ("Streaming")) -> (w446:T8)
            n136 = Wait on Notification(notifier=w440, ignore previous (F)=TRUE, timeout in ms (-1)=w441, error in (no error)=w444) -> (error out=w439:errorcluster)  [unwired: 3 out]
          }
        }
      }
      frame "Exit", Default {
        w454 = FALSE ("force destroy? (F)")
        w460 = TRUE  # Stop Loop?
        w462 = MAG_UI_State."Exit"  # (Value Not Used)
        # "Exit - Exit the application."
        n137 = Release Notifier(notifier=w459, force destroy? (F)=w454, error in (no error)=w456) -> (error out=w458:errorcluster)  [unwired: 2 out]
        n138 = Release Notifier(notifier=w453, force destroy? (F)=w454, error in (no error)=w458) -> (error out=w457:errorcluster)  [unwired: 2 out]
        n139 = Release Notifier(notifier=w452, force destroy? (F)=w454, error in (no error)=w457) -> (error out=w455:errorcluster)  [unwired: 2 out]
      }
    }
    "Status" <- w162
    n140 = Or(x=w166, y=w168) -> (x .or. y?=w167:bool)
  }
  n141 = while {
    shift-right: [w470] -> _
    shift-left: MAG_Display_State."Initialise" -> [w471]
    shift-right: [w466] -> _
    shift-left: _ -> [w469]
    tunnel: w12 -> [w465]
    tunnel: [w464] -> _
    i -> [w463]
    stop <- w467 stop-if-true
    # "Visualisation Loop (Displays Data)"
    n142 = case shown="\"Display\"" w471 {
      tunnel: [MAG_Display_State."Initialise" MAG_Display_State."Display" MAG_Display_State."Display"] -> w470
      tunnel: [w474 FALSE ("Stop Loop?") FALSE ("Stop Loop?")] -> w468
      tunnel: w469 -> [w473 w486 w499]
      tunnel: [w473 w485 w499] -> w466
      tunnel: w465 -> [_ w487 w496]
      tunnel: [_ w484 w496] -> w464
      tunnel: w463 -> [_ _ _]
      frame "Exit", Default {
        w474 = TRUE  # Stop Loop?
        # "Exit - Exit the application."
      }
      frame "Display" {
        n143 = Wait on Notification(notifier=w487, error in (no error)=w486) -> (notifier out=w484:refnum<notifier>, notification=w483:T6, error out=w485:errorcluster)  [unwired: 2 in, 1 out]
        "notification" <- w483
        n144 = Unbundle By Name(w483) -> ("Data"=w475:dbl[][])
        "Sensor Readings" <- w475
        n145 = call "data_grid_v128.vi"("No. Columns"=8, "No. Rows"=16, "Sensor Data"=w475) -> ("Y (GRID)"=w480:dbl[][], "X (GRID)"=w479:dbl[][], "Z (GRID)"=w478:dbl[][], "Mag_GRID"=w482:dbl[][])  [unwired: 5 in]
        n146 = case shown="\"3D\"" "Tab Control" {
          tunnel: w482 -> [w491 _]
          tunnel: w480 -> [_ _]
          tunnel: w479 -> [_ _]
          tunnel: w478 -> [_ w494]
          frame "2D", Default {
            n147 = Index Array(array=w491, index (row)="Node") -> (element=w493:dbl[])  [unwired: 1 in]
            n148 = Array To Cluster(array=w493) -> (cluster=→"Node Response":T15)
          }
          frame "3D" {
            n149 = call <vilib>:"create_plot_surface.vi"("z matrix"=w494) -> ("plots out"=→"3D Graph":refnum<class "Base Datatype.lvclass">[])  [unwired: 4 in, 6 out]
          }
        }
      }
      frame "Initialise" {
      }
    }
    n150 = Or(x=w466, y=w468) -> (x .or. y?=w467:bool)
    "ui" <- w463
  }
  n151 = call <vilib>:"Simple Error Handler.vi"("error in (no error)"=w18) -> ()  [unwired: 4 in, 5 out]
  n152 = Unbundle By Name(w2) -> ("Serial Refnum"=w3:refnum<visa-resource-name>)
  n153 = VISA Clear(VISA resource name=w3, error in (no error)=w1) -> (VISA resource name out=w5:refnum<visa-resource-name>, error out=w4:errorcluster)
  n154 = VISA Close(VISA resource name=w5, error in (no error)=w4) -> ()  [unwired: 1 out]
